vi "MOVE_TAPE_MEASURE.vi"(10 "argv":string[](array[string]), 11 "args":u8) -> ()   [LabVIEW 2014]
uses:
  Robot Global Data.vi
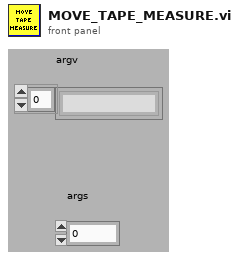
[diagram p1: front panel]
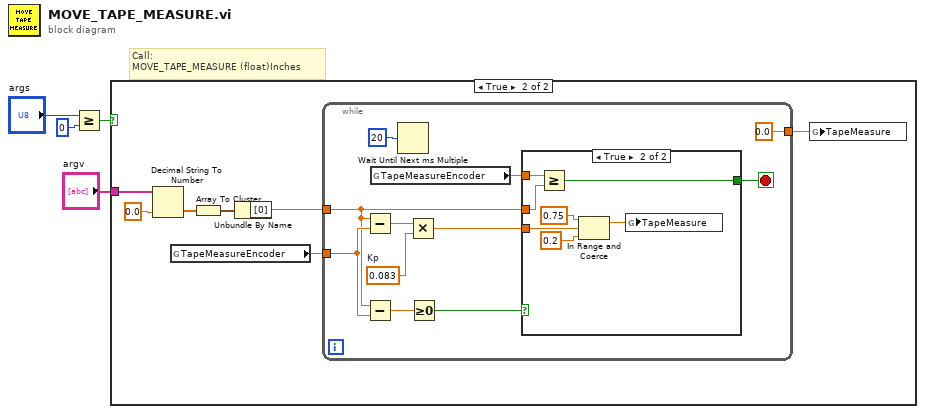
[diagram p0: block diagram]
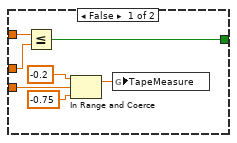
[diagram p3: hidden frame]
diagram:
  # "Call:\nMOVE_TAPE_MEASURE (float)Inches"
  n1 = Greater Or Equal?(x="args", y=u8 0) -> (x >= y?=w4:bool)
  n2 = case shown="True" w4 {
    tunnel: "argv" -> [_ w11]
    frame False {
    }
    frame True {
      n3 = Decimal String To Number(string=w11, default (0L)=0.0 ("default (0 I32)")) -> (number=w9:dbl[])  [unwired: 2 out]
      n4 = global read "Robot Global Data.vi" "TapeMeasureEncoder"() -> (w6:dbl)
      n5 = Array To Cluster(array=w9) -> (cluster=w8:cluster{"[0]":dbl, "[1]":dbl})
      n6 = Unbundle By Name(w8) -> ("[0]"=w5:dbl)
      n7 = while {
        tunnel: [0.0 ("LeftMotorValue")] -> w7
        tunnel: w6 -> [w16]
        tunnel: w5 -> [w12]
        stop <- w20 stop-if-true
        w15 = 0.083  # Kp
        n8 = Subtract(x=w12, y=w16) -> (x-y=w14:dbl)
        n9 = Subtract(x=w12, y=w16) -> (x-y=w17:dbl)
        n10 = global read "Robot Global Data.vi" "TapeMeasureEncoder"() -> (w18:dbl)
        n11 = Wait Until Next ms Multiple(millisecond multiple=u32 20) -> ()  [unwired: 1 out]
        n12 = Multiply(x=w14, y=w15) -> (x*y=w13:dbl)
        n13 = Greater Or Equal To 0?(x=w17) -> (x >= 0?=w21:bool)
        n14 = case shown="True" w21 {
          tunnel: w18 -> [w28 w35]
          tunnel: [w29 w36] -> w20
          tunnel: w12 -> [w27 w34]
          tunnel: w13 -> [w26 w33]
          frame False {
            n15 = Less Or Equal?(x=w28, y=w27) -> (x <= y?=w29:bool)
            n16 = In Range and Coerce(upper limit=-0.2, x=w26, lower limit=-0.75) -> (coerced(x)=w25:dbl)  [unwired: 1 out]
            n17 = global write "Robot Global Data.vi" "TapeMeasure"(w25) -> ()
          }
          frame True {
            n18 = Greater Or Equal?(x=w35, y=w34) -> (x >= y?=w36:bool)
            n19 = In Range and Coerce(upper limit=0.75, x=w33, lower limit=0.2) -> (coerced(x)=w32:dbl)  [unwired: 1 out]
            n20 = global write "Robot Global Data.vi" "TapeMeasure"(w32) -> ()
          }
        }
      }
      n21 = global write "Robot Global Data.vi" "TapeMeasure"(w7) -> ()
    }
  }
